vi "Test Populating B line to memory.vi"() -> ()   [LabVIEW 2018]
uses:
  General/Controls/Save Bline to Mem Control.ctl
  General/Controls/System Parameters.ctl
  General/Controls/Optical Parameters.ctl
  General/Controls/Vibratome Parameters.ctl
  General/Controls/Translation Stage Parameters.ctl
  Hardware Mfg/Thorlabs Translation Stages/Controls/Translation Stage Cluster.ctl
  General/Controls/Translation Stage Types.ctl
  General/Controls/Imaging Parameters.ctl
  General/Controls/Scan Direction.ctl
  General/type defines/Alazar parameters.ctl
  Hardware Mfg/AlazarTech SDK/Controls/General Trigger Settings.ctl
  Hardware Mfg/AlazarTech SDK/Controls/Trigger Engine Controls.ctl
  Hardware Mfg/AlazarTech SDK/Controls/Alazar Device ID.ctl
  Hardware Mfg/AlazarTech SDK/Controls/Channel Input Controls.ctl
  Hardware Mfg/AlazarTech SDK/Controls/Alazar Acquisition Settings.ctl
  Hardware Mfg/AlazarTech SDK/Controls/Clock Controls.ctl
  General/type defines/Manual Controls.ctl
  General/type defines/FFT parameters.ctl
  General/type defines/FFT mode.ctl
  General/type defines/Vibratome Param.ctl
panel:
  out "time per Bline":dbl
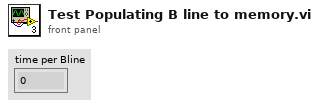
[diagram p1: front panel]
types:
  T1 = typedef "System Parameters.ctl" = cluster{"Optical Parameters":T2, "Vibratome":T3, "Table Stages":T4, "Imaging Parameter":T7, "Galvo HW Parameters":cluster{"Analog Out Channel":tag, "Min Voltage":dbl, "Max Voltage":dbl, "Pixel Clock Source":tag, "Sample Rate":dbl, "Line Clock Out Ch":tag}, "Alazar parameters":T9, "Mosaic Paramter":cluster{"X Axis":cluster{"Start [mm]":dbl, "Steps [pts]":dbl, "End [mm]":dbl}, "Y Axis":cluster{"Start [mm]":dbl, "Steps [pts]":dbl, "End [mm]":dbl}, "Scan Pattern":enum16{"Uni-directional", "Bi-Directional", "Spiral Out", "Spiral In"}, "Overlap Options":cluster{"Overlap Type":enum16{"No Overlap", "X Only", "Y Only", "X and Y"}, "Percent Overlap":u8, "Justify":enum16{"Start", "Center", "End"}}}, "Manual Controls":T16, "Vibratome Axis":T19}
  T2 = typedef "Optical Parameters.ctl" = cluster{"Obj. Focal Length [mm]":dbl, "Scan Lens EFL[mm]":dbl, "Tube Lens EFL[mm]":dbl, "Galvo V Range (+/-)":dbl, "Galvo Max Half Angle [Deg]":dbl, "Max Galvo Range[%]":dbl}
  T3 = typedef "Vibratome Parameters.ctl" = cluster{"Z Bottom [mm]":dbl, "Pre Cut Dwell [s]":dbl, "Blade Frequency [RPM]":u16, "Slice Speed [mm/s]":dbl, "Post Cut Dwell [s]":dbl, "Ramp Time [s]":dbl, "Start X [mm]":dbl, "Start Y [mm]":dbl, "Slice Length [mm]":dbl, "Slice Axis":enum16{"X Axis", "Y Axis", "Z Axis"}, "Controller VISA Ref":refnum<visa-resource-name>}
  T4 = typedef "Translation Stage Parameters.ctl" = cluster{"X Stage":T5, "Y Stage":T5, "Z Stage":T5}
  T5 = typedef "Translation Stage Cluster.ctl" = cluster{"Position":dbl, "Is.Enabled?":bool, "Is.Connected?":bool, "Device SN":string, "AccelerationMaximum":dbl, "VelocityMaximum":dbl, "Acceleration":dbl, "Velocity":dbl, "waitTimeout (ms)":i32, "Model":T6, "Is.Homed?":bool}
  T6 = typedef "Translation Stage Types.ctl" = enum16{"None", "Thorlabs LTS", "Thorlabs MLJ"}
  T7 = typedef "Imaging Parameters.ctl" = cluster{"Raster Scan Direction":T8, "Pixel Dwell Time [Clock Cycles]":u16, "Flyback Time [Clock Cycles]":u16, "XY Center [um]":cluster{"X":dbl, "Y":dbl}, "Pixel Step Size [um]":dbl, "XY Image Size":enum16{"32 x 32", "64 x 64", "128 x 128", "256 x 256", "512 x 512", "1024 x 1024", "2048 x 2048"}, "Custom":bool, "Custom Size":cluster{"X":u16, "Y":u16}, "Line Averages":u8}
  T8 = typedef "Scan Direction.ctl" = enum16{"Uni Directional", "Bi Directional", "None"}
  T9 = typedef "Alazar parameters.ctl" = cluster{"Trigger Settings":cluster{"General Trigger Settings":T10, "Trigger Engine 1":T11, "Trigger Engine 2":T11}, "Device ID":T12, "Ch A Input Control":T13, "Ch B Input Control":T13, "Acq Settings":T14, "Capture Clock":T15}
  T10 = typedef "General Trigger Settings.ctl" = cluster{"Trigger Operation":u32, "Coupling ID":u32, "Range ID":u32, "Delay":u32, "Timeout Ticks":u32, "Mode":u32, "Parameter":u32}
  T11 = typedef "Trigger Engine Controls.ctl" = cluster{"Trigger Engine":u32, "Source":u32, "Slope":u32, "Level":u32}
  T12 = typedef "Alazar Device ID.ctl" = cluster{"System ID":u32, "Board ID":u32}
  T13 = typedef "Channel Input Controls.ctl" = cluster{"Channel":u8, "Coupling":u32, "Range":u32, "Impedance":u32}
  T14 = typedef "Alazar Acquisition Settings.ctl" = cluster{"Record Length":u32, "Offset":u32, "Records Per Buffer":u32, "Records Count (Records/Acq)":u32, "Window Type":u32, "Footer":u32, "Samples per record":u32, "Output Format":u32}
  T15 = typedef "Clock Controls.ctl" = cluster{"Sample Rate":u32, "Decimation":u32, "Source":u32, "Edge":u32}
  T16 = typedef "Manual Controls.ctl" = cluster{"Z0":dbl, "Z0 image":dbl, "Data Path":path, "Save parameters":T17, "Center Galvos":bool, "Acquisition mode":T18, "PSOCT Channel":u32, "Save":bool, "AIP rotation angle":dbl, "Scan Parameters":cluster{"# Scan":cluster{"#Ascan":i32, "#Bscan":i32}, "# Rpt":cluster{"#ARpt":i32, "#BRpt":i32}, "Aline Rate":u16, "# Extra":cluster{"# ARpt_extra":i32, "#Brtn_extra":i32}}, "ROI Parameters":cluster{"ROI (mm)":cluster{"X (mm)":dbl, "Y (mm)":dbl}, "Shift (mm)":cluster{"Xshift (mm)":sgl, "Yshift (mm)":sgl}}, "Objective":u16}
  T17 = typedef "FFT parameters.ctl" = cluster{"start pixel":i32, "#pixels to save":i32}
  T18 = typedef "FFT mode.ctl" = enum16{"ThorOCT B line", "ThorOCT Spectral", "ThorOCT FFT", "Alazar B line", "Alazar FFT", "GPU FFT", "Alazar Spectral"}
  T19 = typedef "Vibratome Param.ctl" = cluster{"Start [mm](Next cut height)":dbl, "thick slice[um]":dbl, "#repitition":u16, "thin slice[um]":dbl, "#thin slices":u16}
  T20 = typedef "Save Bline to Mem Control.ctl" = enum16{"Output data", "Save(ThorOCT)", "Save(PSOCT)", "FFT and Save", "Uninit", "PSOCT Spectral buffer Set", "PSOCT Spatial buffer Set", "PSOCT Spectral buffer Init", "PSOCT Spatial buffer Init", "ThorOCT Spectral buffer Init", "ThorOCT Spatial buffer Init", "ThorOCT Spectral buffer Set", "ThorOCT Spatial buffer Set", "ThorOCT Spectral Save", "Alazar Spectral Save"}
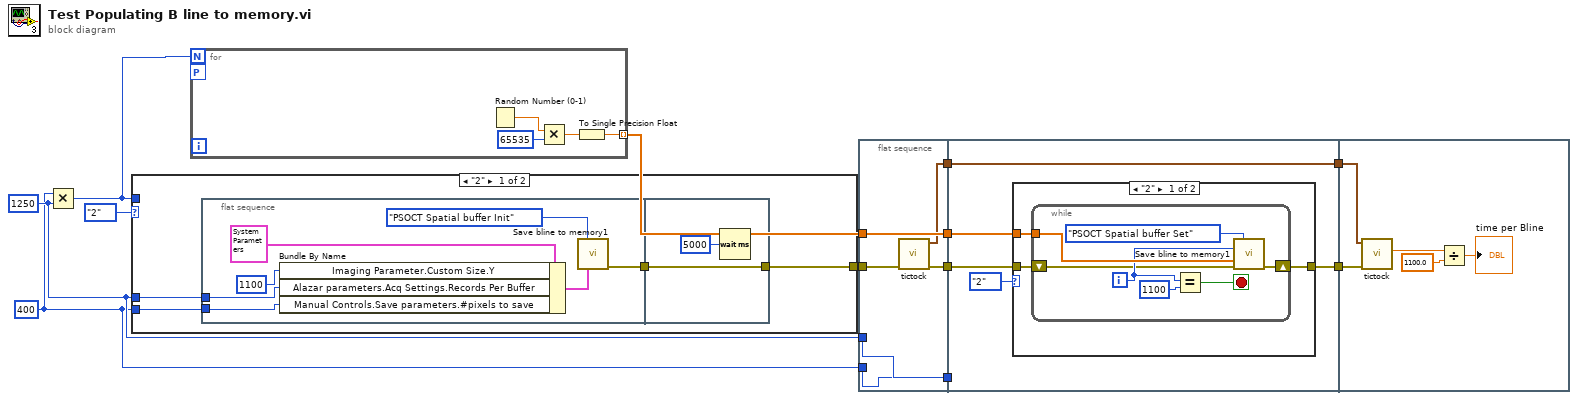
[diagram p0: block diagram]
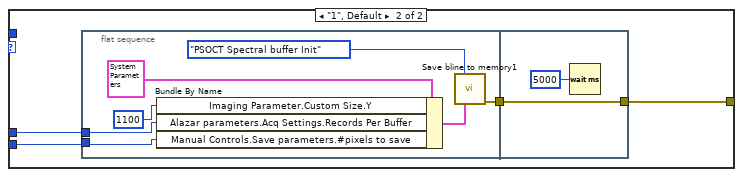
[diagram p2: hidden frame]
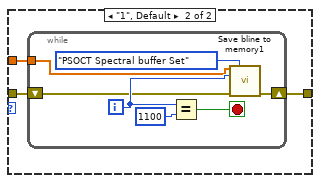
[diagram p3: hidden frame]
diagram:
  w3 = 1250
  w2 = 400
  n1 = Multiply(x=w2, y=w3) -> (x*y=w12:i32)
  n2 = case shown="\"2\"" enum16{"0", "1", "2"}."2" {
    tunnel: w12 -> [_ _]
    tunnel: w3 -> [w17 w30]
    tunnel: w2 -> [w16 w29]
    tunnel: [w15 w28] -> w1
    frame "2" {
      n3 = flat-sequence {
        tunnel: w17 -> [w22]
        tunnel: w16 -> [w21]
        tunnel: [w19] -> w14
        tunnel: [w26] -> w15
        tunnel: w14 -> [w26]
        frame #0 {
          n4 = Bundle By Name(cluster=T1 {"Optical Parameters"={"Obj. Focal Length [mm]"=0.0, "Scan Lens EFL[mm]"=0.0, "Tube Lens EFL[mm]"=0.0, "Galvo V Range (+/-)"=0.0, "Galvo Max Half Angle [Deg]"=0.0, "Max Galvo Range[%]"=0.0}, "Vibratome"={"Z Bottom [mm]"=0.0, "Pre Cut Dwell [s]"=0.0, "Blade Frequency [RPM]"=0, "Slice Speed [mm/s]"=0.0, "Post Cut Dwell [s]"=0.0, "Ramp Time [s]"=0.0, "Start X [mm]"=0.0, "Start Y [mm]"=0.0, "Slice Length [mm]"=0.0, "Slice Axis"=enum."Y Axis", "Controller VISA Ref"="COM4"}, "Table Stages"={"X Stage"={"Position"=0.0, "Is.Enabled?"=FALSE, "Is.Connected?"=FALSE, "Device SN"="45876539", "AccelerationMaximum"=0.0, "VelocityMaximum"=0.0, "Acceleration"=0.0, "Velocity"=0.0, "waitTimeout (ms)"=0, "Model"=enum."None", "Is.Homed?"=FALSE}, "Y Stage"={"Position"=0.0, "Is.Enabled?"=FALSE, "Is.Connected?"=FALSE, "Device SN"="45876539", "AccelerationMaximum"=0.0, "VelocityMaximum"=0.0, "Acceleration"=0.0, "Velocity"=0.0, "waitTimeout (ms)"=0, "Model"=enum."None", "Is.Homed?"=FALSE}, "Z Stage"={"Position"=0.0, "Is.Enabled?"=FALSE, "Is.Connected?"=FALSE, "Device SN"="45876539", "AccelerationMaximum"=0.0, "VelocityMaximum"=0.0, "Acceleration"=0.0, "Velocity"=0.0, "waitTimeout (ms)"=0, "Model"=enum."None", "Is.Homed?"=FALSE}}, "Imaging Parameter"={"Raster Scan Direction"=enum."Bi Directional", "Pixel Dwell Time [Clock Cycles]"=1, "Flyback Time [Clock Cycles]"=0, "XY Center [um]"={"X"=1.0, "Y"=1.0}, "Pixel Step Size [um]"=1.0, "XY Image Size"=enum."256 x 256", "Custom"=FALSE, "Custom Size"={"X"=1, "Y"=1}, "Line Averages"=1}, "Galvo HW Parameters"={"Analog Out Channel"="GalvoCtrl/ao0,GalvoCtrl/ao1", "Min Voltage"=-10.0, "Max Voltage"=10.0, "Pixel Clock Source"="/GalvoCtrl/PFI0", "Sample Rate"=1000.0, "Line Clock Out Ch"="GalvoCtrl/port0/line0"}, "Alazar parameters"={"Trigger Settings"={"General Trigger Settings"={"Trigger Operation"=0, "Coupling ID"=2, "Range ID"=2, "Delay"=0, "Timeout Ticks"=0, "Mode"=1, "Parameter"=1}, "Trigger Engine 1"={"Trigger Engine"=0, "Source"=2, "Slope"=1, "Level"=140}, "Trigger Engine 2"={"Trigger Engine"=1000, "Source"=2048, "Slope"=2048, "Level"=140}}, "Device ID"={"System ID"=1, "Board ID"=1}, "Ch A Input Control"={"Channel"=1, "Coupling"=2, "Range"=10, "Impedance"=2}, "Ch B Input Control"={"Channel"=2, "Coupling"=2, "Range"=10, "Impedance"=2}, "Acq Settings"={"Record Length"=1440, "Offset"=0, "Records Per Buffer"=2048, "Records Count (Records/Acq)"=2147483647, "Window Type"=1, "Footer"=0, "Samples per record"=2048, "Output Format"=257}, "Capture Clock"={"Sample Rate"=100, "Decimation"=0, "Source"=2, "Edge"=0}}, "Mosaic Paramter"={"X Axis"={"Start [mm]"=0.0, "Steps [pts]"=0.0, "End [mm]"=0.0}, "Y Axis"={"Start [mm]"=0.0, "Steps [pts]"=0.0, "End [mm]"=0.0}, "Scan Pattern"=enum."Uni-directional", "Overlap Options"={"Overlap Type"=enum."No Overlap", "Percent Overlap"=0, "Justify"=enum."Start"}}, "Manual Controls"={"Z0"=10.0, "Z0 image"=0.0, "Data Path"=path "", "Save parameters"={"start pixel"=45, "#pixels to save"=100}, "Center Galvos"=FALSE, "Acquisition mode"=enum."Alazar FFT", "PSOCT Channel"=1, "Save"=FALSE, "AIP rotation angle"=0.0, "Scan Parameters"={"# Scan"={"#Ascan"=150, "#Bscan"=400}, "# Rpt"={"#ARpt"=1, "#BRpt"=1}, "Aline Rate"=2, "# Extra"={"# ARpt_extra"=5, "#Brtn_extra"=60}}, "ROI Parameters"={"ROI (mm)"={"X (mm)"=1.0, "Y (mm)"=1.0}, "Shift (mm)"={"Xshift (mm)"=0.0, "Yshift (mm)"=0.0}}, "Objective"=30}, "Vibratome Axis"={"Start [mm](Next cut height)"=45.85, "thick slice[um]"=2.1, "#repitition"=111, "thin slice[um]"=2.1, "#thin slices"=111}} ("System Parameters"), "Imaging Parameter.Custom Size.Y"=u16 1100, "Alazar parameters.Acq Settings.Records Per Buffer"=w22, "Manual Controls.Save parameters.#pixels to save"=w21) -> (w18:T1)
          n5 = call "Save bline to memory1.vi"("action"=Save_Bline_to_Mem_Control."PSOCT Spatial buffer Init", "System Parameters"=w18) -> ("error out"=w19:errorcluster)  [unwired: 13 in]
        }
        frame #1 {
          n6 = Wait (ms)(milliseconds to wait=u32 5000) -> ()  [unwired: 1 out]
        }
      }
    }
    frame "1", Default {
      n7 = flat-sequence {
        tunnel: w30 -> [w35]
        tunnel: w29 -> [w34]
        tunnel: [w32] -> w27
        tunnel: [w39] -> w28
        tunnel: w27 -> [w39]
        frame #0 {
          n8 = Bundle By Name(cluster=T1 {"Optical Parameters"={"Obj. Focal Length [mm]"=0.0, "Scan Lens EFL[mm]"=0.0, "Tube Lens EFL[mm]"=0.0, "Galvo V Range (+/-)"=0.0, "Galvo Max Half Angle [Deg]"=0.0, "Max Galvo Range[%]"=0.0}, "Vibratome"={"Z Bottom [mm]"=0.0, "Pre Cut Dwell [s]"=0.0, "Blade Frequency [RPM]"=0, "Slice Speed [mm/s]"=0.0, "Post Cut Dwell [s]"=0.0, "Ramp Time [s]"=0.0, "Start X [mm]"=0.0, "Start Y [mm]"=0.0, "Slice Length [mm]"=0.0, "Slice Axis"=enum."Y Axis", "Controller VISA Ref"="COM4"}, "Table Stages"={"X Stage"={"Position"=0.0, "Is.Enabled?"=FALSE, "Is.Connected?"=FALSE, "Device SN"="45876539", "AccelerationMaximum"=0.0, "VelocityMaximum"=0.0, "Acceleration"=0.0, "Velocity"=0.0, "waitTimeout (ms)"=0, "Model"=enum."None", "Is.Homed?"=FALSE}, "Y Stage"={"Position"=0.0, "Is.Enabled?"=FALSE, "Is.Connected?"=FALSE, "Device SN"="45876539", "AccelerationMaximum"=0.0, "VelocityMaximum"=0.0, "Acceleration"=0.0, "Velocity"=0.0, "waitTimeout (ms)"=0, "Model"=enum."None", "Is.Homed?"=FALSE}, "Z Stage"={"Position"=0.0, "Is.Enabled?"=FALSE, "Is.Connected?"=FALSE, "Device SN"="45876539", "AccelerationMaximum"=0.0, "VelocityMaximum"=0.0, "Acceleration"=0.0, "Velocity"=0.0, "waitTimeout (ms)"=0, "Model"=enum."None", "Is.Homed?"=FALSE}}, "Imaging Parameter"={"Raster Scan Direction"=enum."Bi Directional", "Pixel Dwell Time [Clock Cycles]"=1, "Flyback Time [Clock Cycles]"=0, "XY Center [um]"={"X"=1.0, "Y"=1.0}, "Pixel Step Size [um]"=1.0, "XY Image Size"=enum."256 x 256", "Custom"=FALSE, "Custom Size"={"X"=1, "Y"=1}, "Line Averages"=1}, "Galvo HW Parameters"={"Analog Out Channel"="GalvoCtrl/ao0,GalvoCtrl/ao1", "Min Voltage"=-10.0, "Max Voltage"=10.0, "Pixel Clock Source"="/GalvoCtrl/PFI0", "Sample Rate"=1000.0, "Line Clock Out Ch"="GalvoCtrl/port0/line0"}, "Alazar parameters"={"Trigger Settings"={"General Trigger Settings"={"Trigger Operation"=0, "Coupling ID"=2, "Range ID"=2, "Delay"=0, "Timeout Ticks"=0, "Mode"=1, "Parameter"=1}, "Trigger Engine 1"={"Trigger Engine"=0, "Source"=2, "Slope"=1, "Level"=140}, "Trigger Engine 2"={"Trigger Engine"=1000, "Source"=2048, "Slope"=2048, "Level"=140}}, "Device ID"={"System ID"=1, "Board ID"=1}, "Ch A Input Control"={"Channel"=1, "Coupling"=2, "Range"=10, "Impedance"=2}, "Ch B Input Control"={"Channel"=2, "Coupling"=2, "Range"=10, "Impedance"=2}, "Acq Settings"={"Record Length"=1440, "Offset"=0, "Records Per Buffer"=2048, "Records Count (Records/Acq)"=2147483647, "Window Type"=1, "Footer"=0, "Samples per record"=2048, "Output Format"=257}, "Capture Clock"={"Sample Rate"=100, "Decimation"=0, "Source"=2, "Edge"=0}}, "Mosaic Paramter"={"X Axis"={"Start [mm]"=0.0, "Steps [pts]"=0.0, "End [mm]"=0.0}, "Y Axis"={"Start [mm]"=0.0, "Steps [pts]"=0.0, "End [mm]"=0.0}, "Scan Pattern"=enum."Uni-directional", "Overlap Options"={"Overlap Type"=enum."No Overlap", "Percent Overlap"=0, "Justify"=enum."Start"}}, "Manual Controls"={"Z0"=10.0, "Z0 image"=0.0, "Data Path"=path "", "Save parameters"={"start pixel"=45, "#pixels to save"=100}, "Center Galvos"=FALSE, "Acquisition mode"=enum."Alazar FFT", "PSOCT Channel"=1, "Save"=FALSE, "AIP rotation angle"=0.0, "Scan Parameters"={"# Scan"={"#Ascan"=150, "#Bscan"=400}, "# Rpt"={"#ARpt"=1, "#BRpt"=1}, "Aline Rate"=2, "# Extra"={"# ARpt_extra"=5, "#Brtn_extra"=60}}, "ROI Parameters"={"ROI (mm)"={"X (mm)"=1.0, "Y (mm)"=1.0}, "Shift (mm)"={"Xshift (mm)"=0.0, "Yshift (mm)"=0.0}}, "Objective"=30}, "Vibratome Axis"={"Start [mm](Next cut height)"=45.85, "thick slice[um]"=2.1, "#repitition"=111, "thin slice[um]"=2.1, "#thin slices"=111}} ("System Parameters"), "Imaging Parameter.Custom Size.Y"=u16 1100, "Alazar parameters.Acq Settings.Records Per Buffer"=w35, "Manual Controls.Save parameters.#pixels to save"=w34) -> (w31:T1)
          n9 = call "Save bline to memory1.vi"("action"=Save_Bline_to_Mem_Control."PSOCT Spectral buffer Init", "System Parameters"=w31) -> ("error out"=w32:errorcluster)  [unwired: 13 in]
        }
        frame #1 {
          n10 = Wait (ms)(milliseconds to wait=u32 5000) -> ()  [unwired: 1 out]
        }
      }
    }
  }
  n11 = for {
    N: w12 -> [_]
    tunnel: [w40] -> w13 mode=indexing
    workers-P: _ -> [_]
    n12 = Random Number (0-1)() -> (number: 0 to 1=w43:dbl)
    n13 = Multiply(x=w43, y=u16 65535) -> (x*y=w41:dbl)
    n14 = To Single Precision Float(number=w41) -> (single precision float=w40:sgl)
  }
  n15 = flat-sequence {
    tunnel: w2 -> [w47]
    tunnel: w3 -> [w48]
    tunnel: w13 -> [w49]
    tunnel: [w49] -> w11
    tunnel: [w48] -> w10
    tunnel: [w47] -> w9
    tunnel: [w46] -> w7
    tunnel: [w45] -> w6
    tunnel: w1 -> [w44]
    tunnel: w11 -> [w54]
    tunnel: w10 -> [_]
    tunnel: w9 -> [_]
    tunnel: [w50] -> w8
    tunnel: w7 -> [w51]
    tunnel: w6 -> [w53]
    tunnel: [w53] -> w5
    tunnel: w8 -> [w79]
    tunnel: w5 -> [w78]
    frame #0 {
      n16 = call "tictock.vi"("error in (no error)"=w44) -> ("error out"=w46:errorcluster, "seconds since 1Jan1904"=w45:timestamp)  [unwired: 8 in, 1 out]
    }
    frame #1 {
      n17 = case shown="\"2\"" enum16{"0", "1", "2"}."2" {
        tunnel: w54 -> [w57 w67]
        tunnel: w51 -> [w56 w66]
        tunnel: [w55 w65] -> w50
        frame "2" {
          n18 = while {
            tunnel: w57 -> [w63]
            shift-right: [w58] -> w55
            shift-left: w56 -> [w59]
            i -> [w62]
            stop <- w60 stop-if-true
            n19 = Equal?(x=w62, y=1100) -> (x = y?=w60:bool)
            n20 = call "Save bline to memory1.vi"("action"=Save_Bline_to_Mem_Control."PSOCT Spatial buffer Set", "index (row)"=w62, "PSOCT Spatial Bline"=w63, "error in"=w59) -> ("error out"=w58:errorcluster)  [unwired: 11 in]
          }
        }
        frame "1", Default {
          n21 = while {
            tunnel: w67 -> [w68]
            shift-right: [w69] -> w65
            shift-left: w66 -> [w70]
            i -> [w73]
            stop <- w71 stop-if-true
            n22 = Equal?(x=w73, y=1100) -> (x = y?=w71:bool)
            n23 = call "Save bline to memory1.vi"("PSOCTSpectral Bline"=w68, "action"=Save_Bline_to_Mem_Control."PSOCT Spectral buffer Set", "index (row)"=w73, "error in"=w70) -> ("error out"=w69:errorcluster)  [unwired: 11 in]
          }
        }
      }
    }
    frame #2 {
      n24 = call "tictock.vi"("error in (no error)"=w79, "seconds since 1Jan1904 2"=w78) -> ("Numeric"=w77:dbl)  [unwired: 7 in, 2 out]
      n25 = Divide(x=w77, y=1100.0) -> (x/y=→"time per Bline":dbl)
    }
  }
